vi "transmitRFID small_cw.vi"() -> ()   [LabVIEW 2015]
uses:
  <instrlib>/niUSRP/niUSRP Write Tx Data (CDB).vi
panel:
  out "ACK Entered":bool
  out "RFID Pushed":bool
  out "error out":errorcluster
  in  "Parameters Query":T1 {"Session" items=["S0", "S1", "S2", "S3"]; "Sel" items=["All", "All2", "~SL", "SL"]; "M" items=["M=1", "M=2", "M=4", "M=8"]}
  out "Waveform Magnitude":dbl[](graph)
  out "Loop":i32
  in  "Symbol Rate [Hz]":dbl=500000.0 format="%#_13p"
  in  "Parameters Select":T2={"Target"=7, "Action"=0, "MemBank"=1, "truncate"=FALSE} {"MemBank" items=["00 RFU", "01 EPC", "10 TID", "11 User"]; "Action" items=["000", "001", "010", "011", "100", "101", "110", "111"]; "Target" items=["000 Inventoried (S0)", "001 Inventoried (S1)", "010 Inventoried (S2)", "011 Inventoried (S3)", "100 SL", "101 RFU", "110 RFU", "111 RFU"]}
  in  "Parameters Symbols":T3={"Tari"=8e-06, "PW"=0.5, "factor for \"1\" symbol"=0.5, "RTcal"=2.5, "TRcal"=3.0, "Delimiter"=1.25e-05} {"TRcal" min=1.1 max=3.0 step=0.1; "RTcal" min=2.5 max=3.0 step=0.1; "factor for \"1\" symbol" min=0.5 max=1.0 step=0.1; "PW" min=0.265 max=0.525 step=0.001; "Tari" format="%#_3p"}
  out "coerced IQ rate":dbl=100000.0 format="%#_6p"
  out "carrier frequency":dbl=100000.0 format="%#_6p"
  out "coerced gain":dbl format="%#_6f"
  in  "stop":bool
  in  "IQ rate":dbl=2000000.0 format="%#_6p"
  in  "carrier frequency":dbl=920000000.0 format="%#_6p"
  in  "gain":dbl format="%#_6f"
  in  "tx device names":refnum<k15>="192.168.20.13"
  # "Transmit RFID"
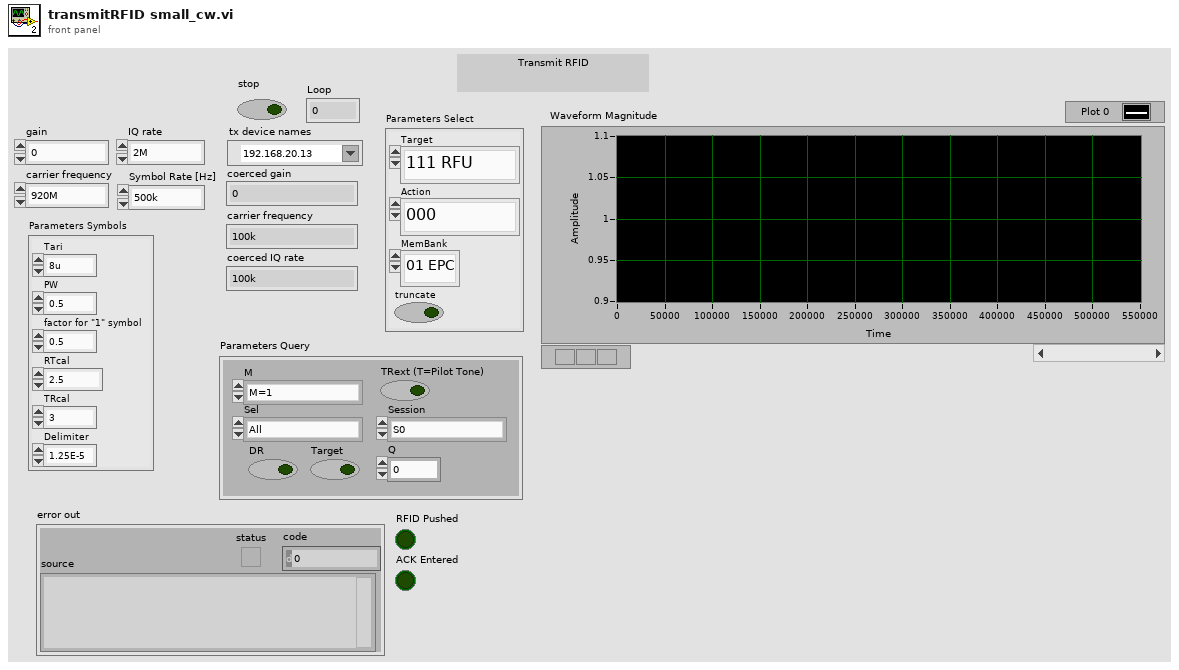
[diagram p1: front panel]
types:
  T1 = cluster{"DR":bool, "M":u16, "TRext (T=Pilot Tone)":bool, "Sel":u16, "Session":u16, "Q":u8, "Target":bool}
  T2 = cluster{"Target":u16, "Action":u16, "MemBank":u16, "truncate":bool}
  T3 = cluster{"Tari":dbl, "PW":dbl, "factor for \"1\" symbol":dbl, "RTcal":dbl, "TRcal":dbl, "Delimiter":dbl}
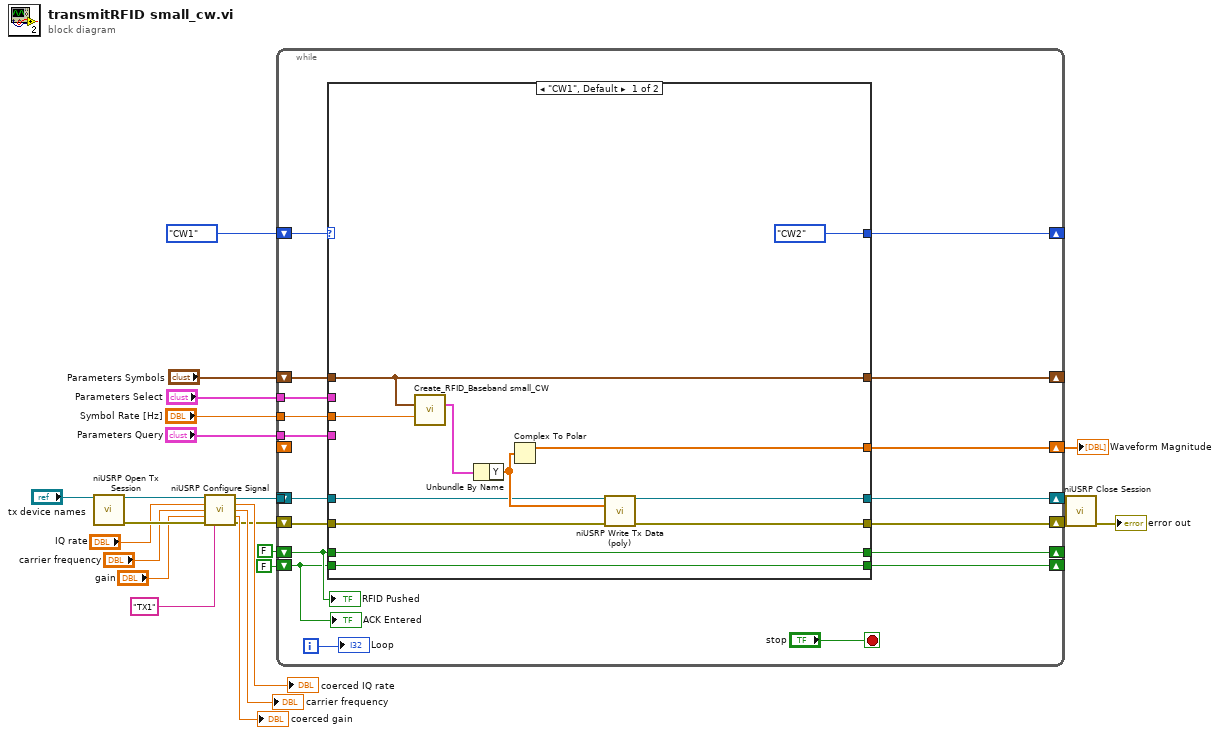
[diagram p0: block diagram]
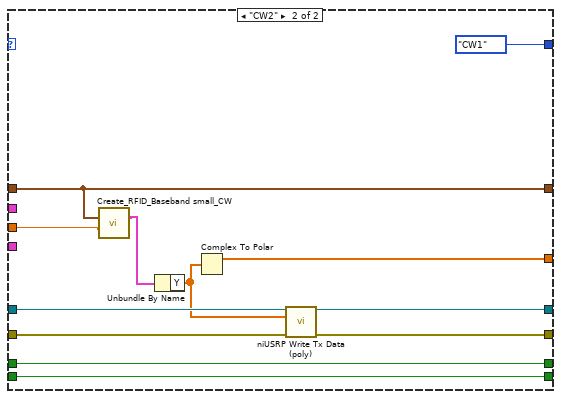
[diagram p2: hidden frame]
diagram:
  n1 = call <instrlib>:"niUSRP Open Tx Session.vi"("device names"="tx device names") -> ("session handle out"=w11:refnum<k15>, "error out"=w23:errorcluster)  [unwired: 13 in]
  n2 = call <instrlib>:"niUSRP Configure Signal.vi"("session handle"=w11, "IQ rate"="IQ rate", "carrier frequency"="carrier frequency", "gain"="gain", "error in (no error)"=w23, "active antenna"="TX1") -> ("session handle out"=w9:refnum<k15>, "coerced IQ rate"=→"coerced IQ rate":dbl, "coerced carrier frequency"=→"carrier frequency":dbl, "coerced gain"=→"coerced gain":dbl, "error out"=w8:errorcluster)  [unwired: 5 in]
  n3 = while {
    tunnel: "Parameters Select" -> [w34]
    tunnel: "Parameters Query" -> [w32]
    tunnel: w9 -> [w39]
    shift-right: [w37] -> w7
    shift-left: w8 -> [w38]
    shift-right: [w36] -> w5
    shift-left: _ -> [_]
    shift-right: [w24] -> _
    shift-left: enum16{"CW1", "CW2"}."CW1" -> [w40]
    shift-right: [w31] -> _
    shift-left: "Parameters Symbols" -> [w35]
    shift-right: [w29] -> _
    shift-left: FALSE -> [w28]
    shift-right: [w27] -> _
    shift-left: FALSE -> [w26]
    shift-right: [w25] -> w1
    shift-left: _ -> [_]
    tunnel: "Symbol Rate [Hz]" -> [w33]
    i -> [w41]
    stop <- "stop" stop-if-true
    n4 = case shown="\"CW1\", Default" w40 {
      tunnel: w39 -> [w52 w65]
      tunnel: w38 -> [w51 w64]
      tunnel: [w50 w63] -> w37
      tunnel: [w49 w62] -> w36
      tunnel: w35 -> [w45 w60]
      tunnel: w34 -> [_ _]
      tunnel: w33 -> [w44 w59]
      tunnel: w32 -> [_ _]
      tunnel: [w45 w60] -> w31
      tunnel: [w48 w54] -> w29
      tunnel: w28 -> [w48 w54]
      tunnel: [w47 w61] -> w27
      tunnel: w26 -> [w47 w61]
      tunnel: [w46 w56] -> w25
      tunnel: [enum16{"CW1", "CW2"}."CW2" enum16{"CW1", "CW2"}."CW1"] -> w24
      frame "CW1", Default {
        n5 = call "Create_RFID_Baseband small_CW.vi"("Parameters Symbols"=w45, "Symbol Rate [Hz]"=w44) -> ("complex waveform"=w43:cluster{"t0":dbl, "dt":dbl, "Y":cdb[]})  [unwired: 12 in, 1 out]
        n6 = Unbundle By Name(w43) -> ("Y"=w53:cdb[])
        n7 = Complex To Polar(r * e^(i*theta)=w53) -> (r=w46:dbl[])  [unwired: 1 out]
        n8 = call-poly <instrlib>:"niUSRP Write Tx Data (poly).vi"("session handle"=w52, "data"=w53, "error in (no error)"=w51) -> ("session handle out"=w49:refnum<k15>, "error out"=w50:errorcluster)  [unwired: 11 in]
      }
      frame "CW2" {
        n9 = call "Create_RFID_Baseband small_CW.vi"("Parameters Symbols"=w60, "Symbol Rate [Hz]"=w59) -> ("complex waveform"=w58:cluster{"t0":dbl, "dt":dbl, "Y":cdb[]})  [unwired: 12 in, 1 out]
        n10 = Unbundle By Name(w58) -> ("Y"=w57:cdb[])
        n11 = Complex To Polar(r * e^(i*theta)=w57) -> (r=w56:dbl[])  [unwired: 1 out]
        n12 = call-poly <instrlib>:"niUSRP Write Tx Data (poly).vi"("session handle"=w65, "data"=w57, "error in (no error)"=w64) -> ("session handle out"=w62:refnum<k15>, "error out"=w63:errorcluster)  [unwired: 11 in]
      }
    }
    "Loop" <- w41
    "RFID Pushed" <- w28
    "ACK Entered" <- w26
  }
  "Waveform Magnitude" <- w1
  n13 = call <instrlib>:"niUSRP Close Session.vi"("session handle"=w5, "error in (no error)"=w7) -> ("error out"=→"error out":errorcluster)  [unwired: 13 in]
